vi "baseline.vi"(0 "N":i32, 1 "X coord profile":dbl[](array[numeric]), 2 "calibration":dbl=0.094, 5 "New Image":T2, 7 "Session Out":T1, 9 "error out":errorcluster, 11 "rectangle selection":i32[](array[numeric]), 12 "k voulue (pN/nm)":dbl=1.0, 13 "longueur fit (pts)":i32=11) -> (4 "baseline":dbl caption="moyenne" format="%0.2f", 6 "sd":dbl caption="écart-type" format="%0.2f", 8 "Image Out":T2, 10 "Session Out 2":T1 caption="Session Out", 15 "error out 2":errorcluster)   [LabVIEW 2017]
uses:
  <vilib>/vision/Image Controls.llb/IMAQ Image.ctl
  <vilib>/userdefined/High Color/IMAQdx.ctl
  <vilib>/vision/driver/IMAQdx.llb/IMAQdx Buffer Number Mode.ctl
  <vilib>/vision/driver/NI_Vision_Acquisition_Software.lvlib
  <resource>/objmgr/imaqdx.rc
  <vilib>/vision/NI_Vision_Development_Module.lvlib
  <vilib>/Analysis/NI_AALPro.lvlib
  <vilib>/Analysis/NI_AALBase.lvlib
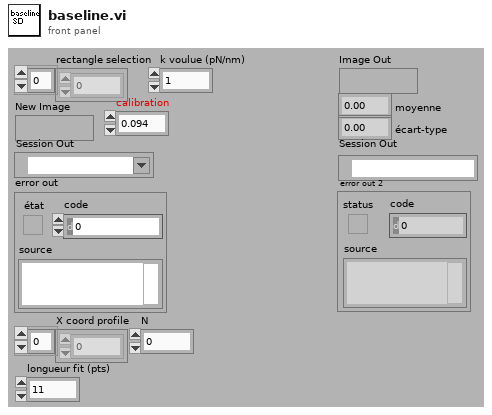
[diagram p1: front panel]
types:
  T1 = typedef "IMAQdx.ctl" = refnum<k21>
  T2 = typedef "IMAQ Image.ctl" = refnum<image>
  T3 = typedef "NI_Vision_Acquisition_Software.lvlib/IMAQdx Buffer Number Mode.ctl" = enum32{"Next", "Last", "Buffer Number", "Every", "Last New"}
  T4 = enum32{"SVD", "Givens", "Givens2", "Householder", "LU Decomposition", "Cholesky"}
  T5 = cluster{"Polynomial Coefficients[0]":dbl, "Polynomial Coefficients[1]":dbl, "Polynomial Coefficients[2]":dbl, "Polynomial Coefficients[3]":dbl, "Polynomial Coefficients[4]":dbl, "Polynomial Coefficients[5]":dbl, "Polynomial Coefficients[6]":dbl, "Polynomial Coefficients[7]":dbl, "Polynomial Coefficients[8]":dbl}
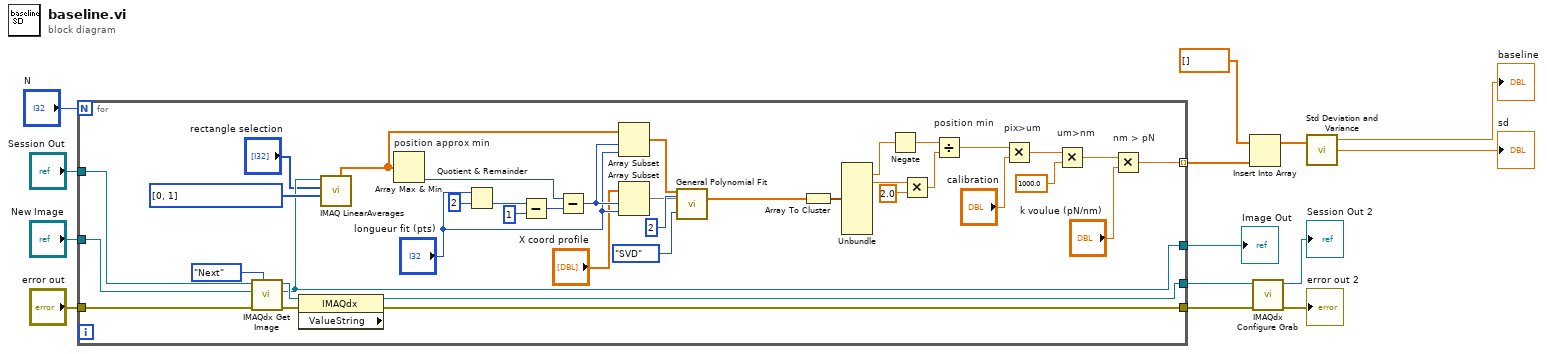
[diagram p0: block diagram]
diagram:
  n1 = for {
    N: "N" -> [_]
    tunnel: "error out" -> [w32]
    tunnel: "Session Out" -> [w24]
    tunnel: [w31] -> w10
    tunnel: [w30] -> w9
    tunnel: [w25] -> w13 mode=indexing
    tunnel: "New Image" -> [w23]
    tunnel: [w21] -> w11
    w37 = i32[] [0, 1] items=["X Axis Averages", "Y Axis Averages", "X + Y Axis Averages", "X - Y Axis Averages"] ("Averages")
    n2 = call <vilib>:"IMAQdx Get Image.vi"("Buffer Number Mode (Next)"=IMAQdx_Buffer_Number_Mode."Next", "error in"=w32, "Image In"=w23, "Session In"=w24) -> ("error out"=w34:errorcluster, "Image Out"=w21:T2, "Session Out"=w22:T1)  [unwired: 1 in, 4 out]
    n3 = property class="IMAQdx" props=["ValueString"](reference=w22, error in=w34) -> (reference out=w30:T1, error out=w31:errorcluster)  [unwired: 1 out]
    n4 = call "IMAQ LinearAverages"("Averages"=w37, "Optional Rectangle"="rectangle selection", "Image Src"=w21) -> ("X Axis Averages"=w36:sgl[])  [unwired: 1 in, 7 out]
    n5 = Array Max & Min "position approx min"(array=w36) -> (min index (indices)=w50:i32)  [unwired: 3 out]
    n6 = Quotient & Remainder(x="longueur fit (pts)", y=2) -> (floor(x/y)=w52:i32)  [unwired: 1 out]
    n7 = Subtract(x=w52, y=1) -> (x-y=w49:i32)
    n8 = Subtract(x=w50, y=w49) -> (x-y=w48:i32)
    n9 = Array Subset(array=w36, index=w48, length="longueur fit (pts)") -> (w35:sgl[])
    n10 = Array Subset(array="X coord profile", index=w48, length="longueur fit (pts)") -> (w20:dbl[])
    n11 = call <vilib>:"General Polynomial Fit.vi"("Y"=w35, "polynomial order"=2, "X"=w20, "algorithm"=T4."SVD") -> ("Polynomial Coefficients"=w44:dbl[])  [unwired: 8 in, 3 out]
    n12 = Array To Cluster(array=w44) -> (cluster=w43:T5)
    n13 = Unbundle(w43) -> ("Polynomial Coefficients[1]"=w42:dbl, "Polynomial Coefficients[2]"=w38:dbl)  [unwired: 7 out]
    n14 = Negate(x=w42) -> (-x=w41:dbl)
    n15 = Multiply(x=w38, y=2.0) -> (x*y=w40:dbl)
    n16 = Divide "position min"(x=w41, y=w40) -> (x/y=w26:dbl)
    n17 = Multiply "pix>um"(x=w26, y="calibration") -> (x*y=w28:dbl)
    n18 = Multiply "um>nm"(x=w28, y=1000.0) -> (x*y=w29:dbl)
    n19 = Multiply "nm > pN"(x=w29, y="k voulue (pN/nm)") -> (x*y=w25:dbl)
  }
  "Image Out" <- w11
  n20 = Insert Into Array(array=dbl[] [] ("tableau"), new element=w13) -> (w12:dbl[])  [unwired: 1 in]
  n21 = call <vilib>:"IMAQdx Configure Grab.vi"("error in"=w10, "Session In"=w9) -> ("error out"=→"error out 2":errorcluster, "Session Out"=→"Session Out 2":T1)  [unwired: 1 in, 7 out]
  n22 = call <vilib>:"Std Deviation and Variance.vi"("X"=w12) -> ("mean"=→"baseline":dbl, "standard deviation"=→"sd":dbl)  [unwired: 1 in, 1 out]
